vi "Eth Status Read status.vi"(7 "Status Reference":T2, 8 "error in (no error)":errorcluster, 11 "N":i32) -> (0 "error out":errorcluster, 1 "status":T1=enum."requests")   [LabVIEW 2019, in "Eth Status.lvlib"]
uses:
  Eth Status.lvlib
  Ctl/ICPCON Status.ctl
  MB_TCP2/MB_TCP_State.ctl
  MB_TCP2/MB_TCP.lvclass
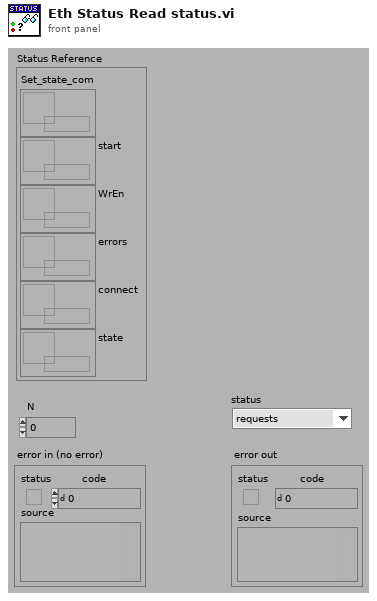
[diagram p1: front panel]
types:
  T1 = typedef "MB_TCP.lvclass/MB_TCP_State.ctl" = enum8{"initialization", "redefine", "standby", "connect", "wait to reconnect", "wait to reset timeout", "configure", "requests", "close connection", "stop"}
  T2 = typedef "Eth Status.lvlib/ICPCON Status.ctl" = cluster{"Set_state_com":refnum<data-value>, "start":refnum<data-value>, "WrEn":refnum<data-value>, "errors":refnum<data-value>, "connect":refnum<data-value>, "state":refnum<data-value>}
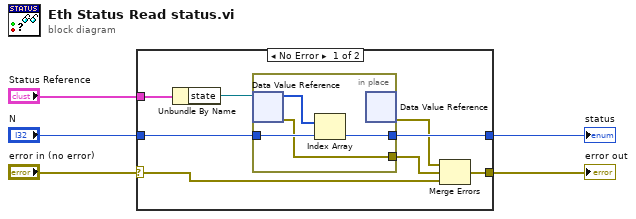
[diagram p0: block diagram]
diagram:
  n1 = case shown="No Error" "error in (no error)" {
    selector: "error in (no error)" -> [w6 w18]
    tunnel: [w10 w18] -> w1
    tunnel: [w13 _] -> w2
    tunnel: "N" -> [w12 _]
    tunnel: "Status Reference" -> [w11 _]
    frame No Error {
      n2 = Unbundle By Name(w11) -> ("state"=w7:refnum<data-value>)
      n3 = in-place {
        in-place-border: w12 -> [w17]
        in-place-border: [w15] -> w13
        in-place-border: [w14] -> w8
        n4 = in-place-dvr #1(w7) -> (w16:T1[], w14:errorcluster)
        n5 = Index Array(array=w16, index=w17) -> (element=w15:T1)
        n6 = in-place-dvr #1() -> (w9:errorcluster)  [unwired: 1 in, 1 out]
      }
      n7 = Merge Errors(w9, w8, w6) -> (w10:errorcluster)
    }
    frame Error {
    }
  }
  "error out" <- w1
  "status" <- w2
